vi "帶青蛙飛吧.vi"(2 "Numeric":i32) -> (3 "英勇的挑戰者請輸入名稱: 2":string)   [LabVIEW 2014]
panel:
  in  "?":bool
  in  "英勇的挑戰者請輸入名稱:":string
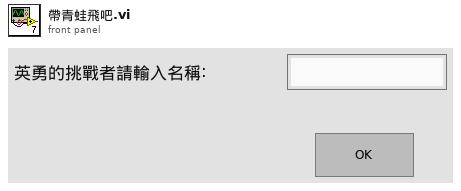
[diagram p1: front panel]
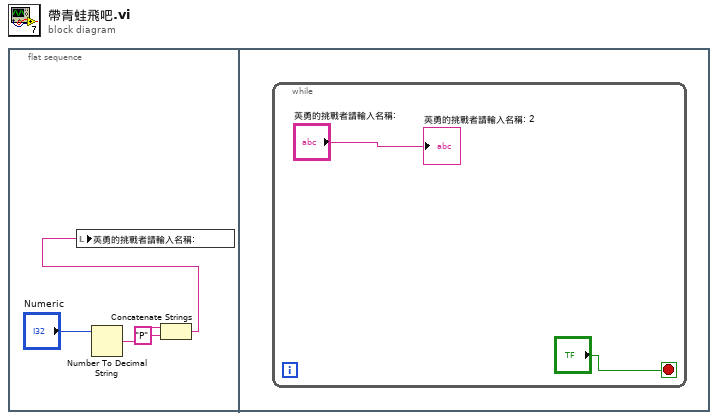
[diagram p0: block diagram]
diagram:
  n1 = flat-sequence {
    frame #0 {
      n2 = Number To Decimal String(number="Numeric") -> (decimal integer string=w3:string)  [unwired: 1 in]
      n3 = Concatenate Strings(w3, "P" ("string")) -> (w1:string)
      n4 = local write "英勇的挑戰者請輸入名稱:"(w1) -> ()
    }
    frame #1 {
      n5 = while {
        stop <- "?" stop-if-true
        "英勇的挑戰者請輸入名稱: 2" <- "英勇的挑戰者請輸入名稱:"
      }
    }
  }
